vi "FPGA - On Delete (Local).vi"(6 "All deleted Refs":T1[](array[typedef]) format="%.0x", 8 "error in (no error)":errorcluster, 11 "Item Ref in":T1 format="%.0x") -> (0 "error out":errorcluster, 3 "Item Ref out":T1 format="%.0x")   [LabVIEW 2016, in "Scan Engine Custom Device.lvlib"]
uses:
  Scan Engine Custom Device.lvlib
  Type Defs/Host - FPGAScanInterfaceMode.ctl
  <vilib>/NI Veristand/Custom Device API/Custom Device Item Ref.ctl
  <vilib>/NI Veristand/Custom Device API/Custom Device API.lvlib
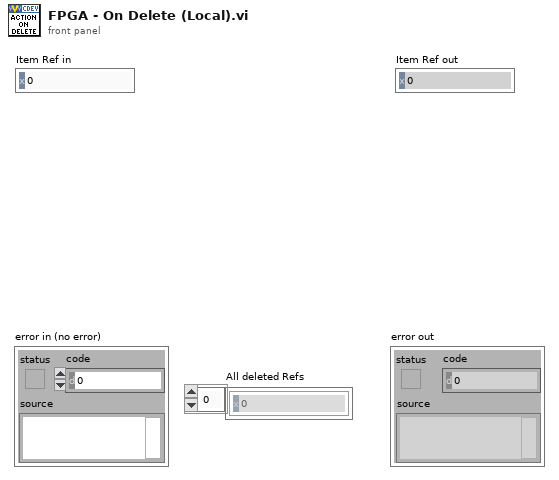
[diagram p1: front panel]
types:
  T1 = typedef "Custom Device API.lvlib/Custom Device Item Ref.ctl" = u64
  T2 = typedef "Scan Engine Custom Device.lvlib/Host - FPGAScanInterfaceMode.ctl" = enum16{"Use Current", "FPGA", "Scan Mode"}
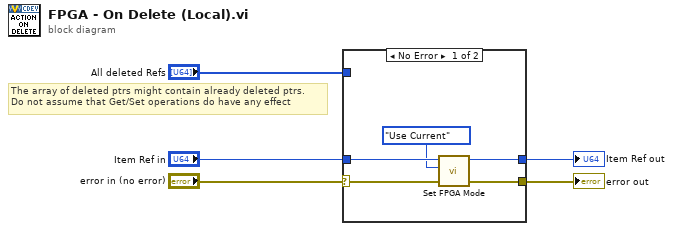
[diagram p0: block diagram]
diagram:
  # "The array of deleted ptrs might contain already deleted ptrs.\nDo not assume that Get/Set operations do have any effect"
  n1 = case shown="No Error" "error in (no error)" {
    selector: "error in (no error)" -> [w9 w12]
    tunnel: [w7 w12] -> w4
    tunnel: "Item Ref in" -> [w10 w11]
    tunnel: [w8 w11] -> w2
    tunnel: "All deleted Refs" -> [_ _]
    frame No Error {
      n2 = call "Set FPGA Mode.vi"("error in (no error)"=w9, "FPGAScanInterfaceMode"=Host_-_FPGAScanInterfaceMode."Use Current", "Item Ref in"=w10) -> ("error out"=w7:errorcluster, "Item Ref out"=w8:T1)  [unwired: 7 in]
    }
    frame Error {
    }
  }
  "error out" <- w4
  "Item Ref out" <- w2
